vi "MDF4 Get DLL Path.vi"(8 "error in (no error)":errorcluster, 10 "Init":bool, 11 "DLL Path":path=path "C:/Users/Hovhannes/Downloads/WriterExample/Debug/WriterExample.exe") -> (0 "error out":errorcluster, 3 "DLL Path Out":path)   [LabVIEW 2019, in "MD4Logger Engine.lvlib"]
uses:
  MD4Logger Engine.lvlib
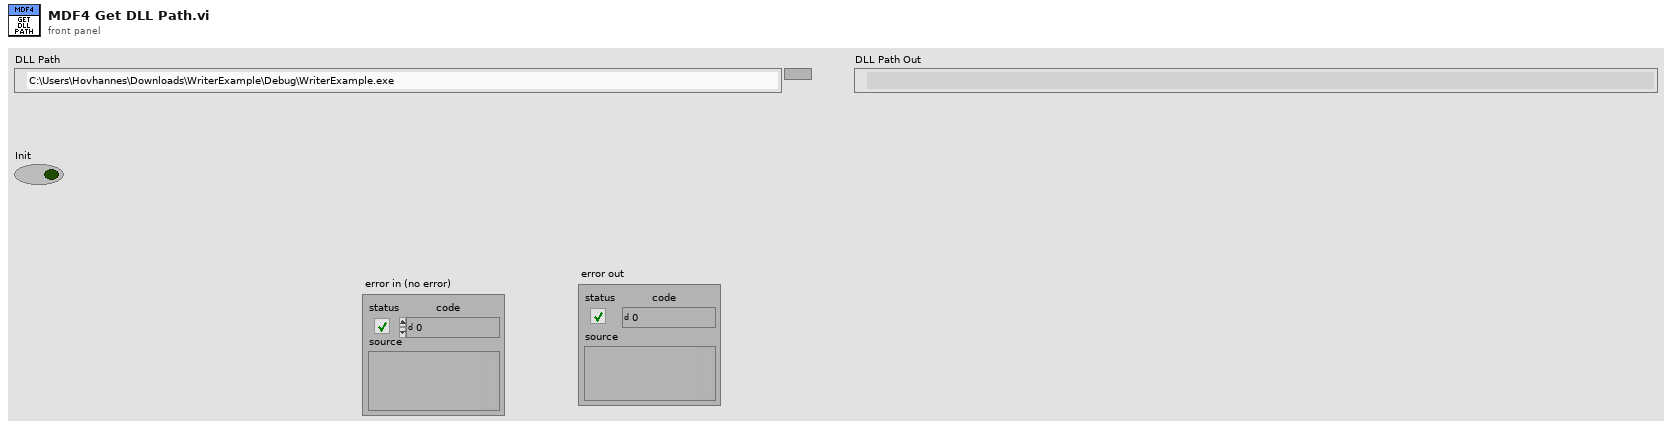
[diagram p1: front panel]
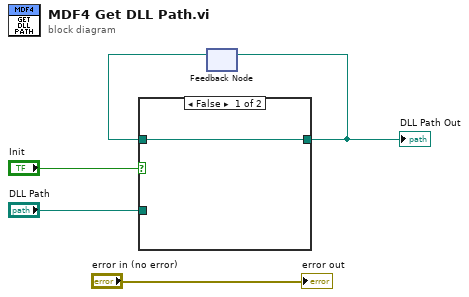
[diagram p0: block diagram]
diagram:
  n1 = feedback #1() -> (w3:path)  [unwired: 1 in]
  n2 = case shown="False" "Init" {
    tunnel: [w6 w7] -> w2
    tunnel: "DLL Path" -> [_ w7]
    tunnel: w3 -> [w6 _]
    frame False {
    }
    frame True {
    }
  }
  "DLL Path Out" <- w2
  n3 = feedback-in #1(w2) -> ()
  "error out" <- "error in (no error)"
